vi "Wave Display UI.vi"() -> ()   [LabVIEW 2016]
uses:
  Architecture/Queue Management/ARC_Queue Create_Single.vi
  Architecture/Queue Management/ARC_Queue Valid.vi
  Architecture/Queue Management/ARC_Queue Destroy_Single.vi
panel:
  out "UnitNo.":i32
  out "波形图":dbl[][](graph)
  in  "Parameter":cluster{"Q-Local":string, "Variant":variant}
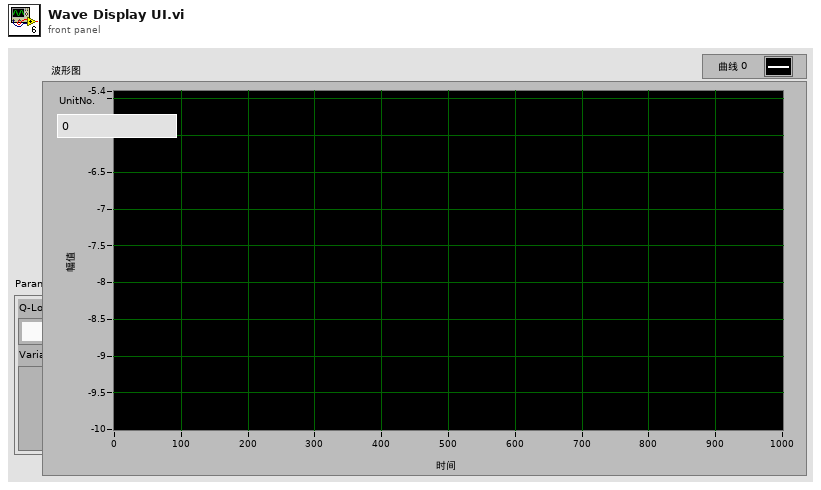
[diagram p1: front panel]
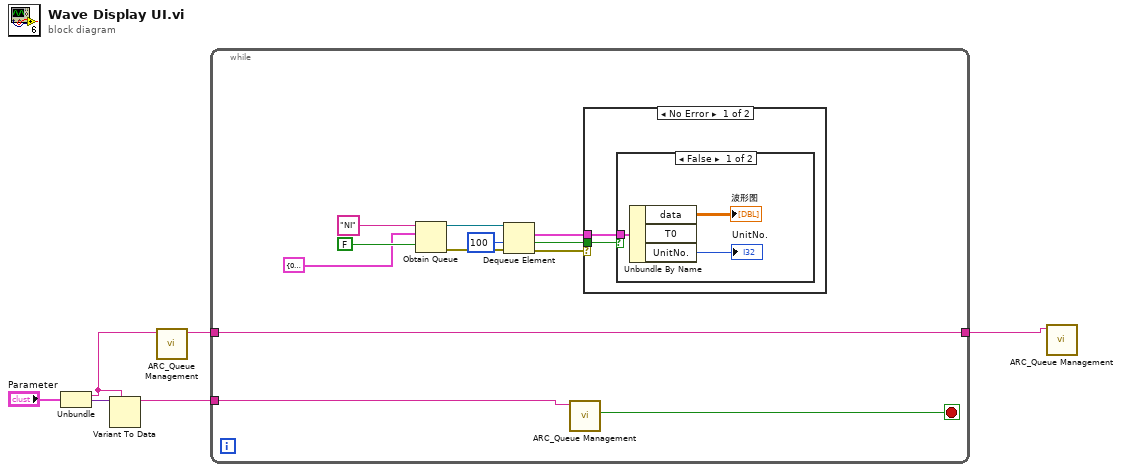
[diagram p0: block diagram]
diagram:
  n1 = Unbundle("Parameter") -> ("Q-Local"=w2:string, "Variant"=w5:variant)
  n2 = Variant To Data(type=w2, Variant=w5) -> (data=w1:string)  [unwired: 1 in, 1 out]
  n3 = call-poly "ARC_Queue Management.vi"("Queue Name"=w2) -> ("Queue Name dup"=w4:string)  [unwired: 8 in, 2 out]
  n4 = while {
    tunnel: w1 -> [w8]
    tunnel: w4 -> [w7]
    tunnel: [w7] -> w3
    stop <- w9 stop-if-true
    n5 = Obtain Queue(name (unnamed)="NI" ("名称（未命名）"), element data type=cluster{"UnitNo.":i32, "data":dbl[][], "T0":dbl} {"UnitNo."=0, "data"=[], "T0"=0.0}, create if not found? (T)=FALSE ("如未找到则创建？(T)")) -> (queue out=w18:refnum<queue>, error out=w17:errorcluster)  [unwired: 2 in, 1 out]
    n6 = Dequeue Element(queue=w18, timeout in ms (-1)=100 ("超时毫秒(-1)"), error in (no error)=w17) -> (element=w10:cluster{"UnitNo.":i32, "data":dbl[][], "T0":dbl}, timed out?=w12:bool, error out=w11:errorcluster)  [unwired: 1 out]
    n7 = call-poly "ARC_Queue Management.vi"("Queue Name(unamed)"=w8) -> ("Not Exist?"=w9:bool)  [unwired: 8 in, 2 out]
    n8 = case shown="No Error" w11 {
      tunnel: w12 -> [w20 _]
      tunnel: w10 -> [w19 _]
      frame No Error {
        n9 = case shown="False" w20 {
          tunnel: w19 -> [w23 _]
          frame False {
            n10 = Unbundle By Name(w23) -> ("data"=→"波形图":dbl[][], "UnitNo."=→"UnitNo.":i32)  [unwired: 1 out]
          }
          frame True {
          }
        }
      }
      frame Error {
      }
    }
  }
  n11 = call-poly "ARC_Queue Management.vi"("Queue Name(unamed)"=w3) -> ()  [unwired: 8 in, 3 out]
